vi "Configure Burst.vi"(0 "VISA resource name":refnum<visa-resource-name>, 1 "Start Phase (0.0 degrees)":dbl=0.002 min=0.0 max=360.0 format="%#.1g", 2 "Burst Cycle (0: N-Cycle)":u16(ring) items=["N-Cycle", "Infinite"], 3 "Number of Cycles (1)":i32=1, 4 "Burst Delay (1.352 μs)":dbl=1.352e-06, 5 "error in (no error)":errorcluster, 6 "Trigger Source (0: Internal)":u16(ring) items=["Internal", "External", "Manual"], 7 "External Trigger Condition (0: Rise)":u16(ring) items=["Rise", "Fall"], 8 "Enable Burst Mode (T:Enable)":bool=TRUE, 9 "Burst Period (0.01 s)":dbl=0.01 format="%#.3g", 10 "Channel (1:Channel 1)":i32(ring)=1 items=["Channel 1"=1, "Channel 2"=2], 11 "Trigger Out Mode (0: Off)":u16(ring) items=["Off", "Rise", "Fall"]) -> (14 "VISA resource name out":refnum<visa-resource-name>, 19 "error out":errorcluster)   [LabVIEW 2023, in "Siglent SDG X Series.lvlib"]
doc: "Configures and enables burst output mode.\n\nNote: Burst mode is not available for noise waveform."
uses:
  Siglent SDG X Series.lvlib
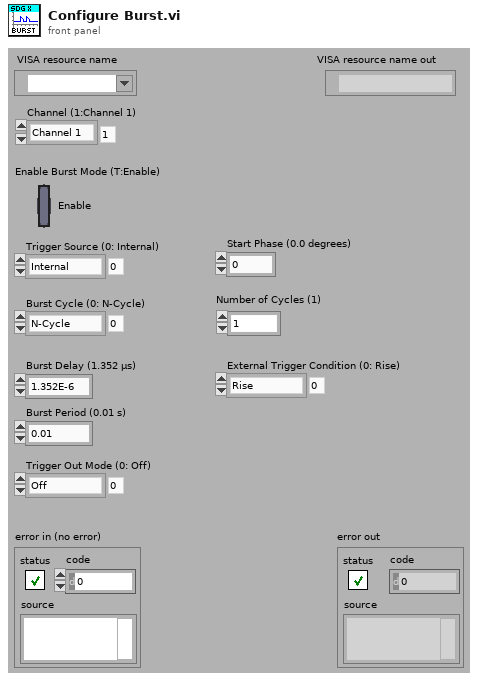
[diagram p1: front panel]
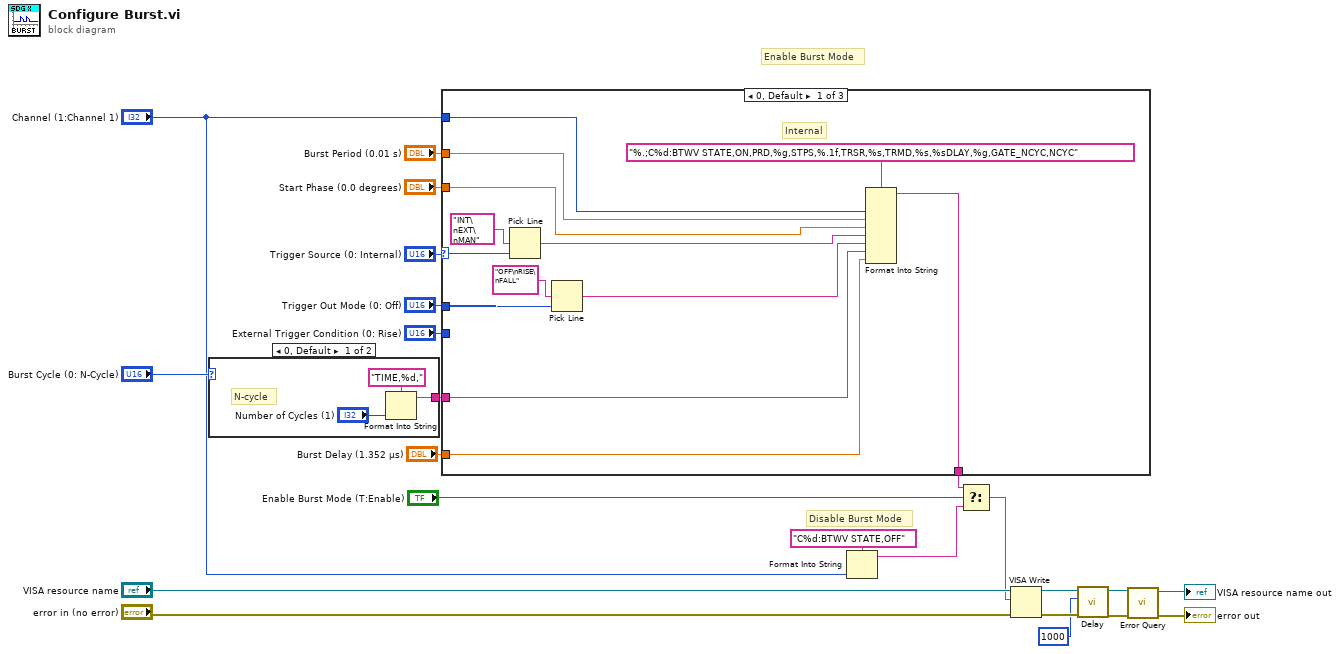
[diagram p0: block diagram]
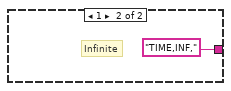
[diagram p2: hidden frame]
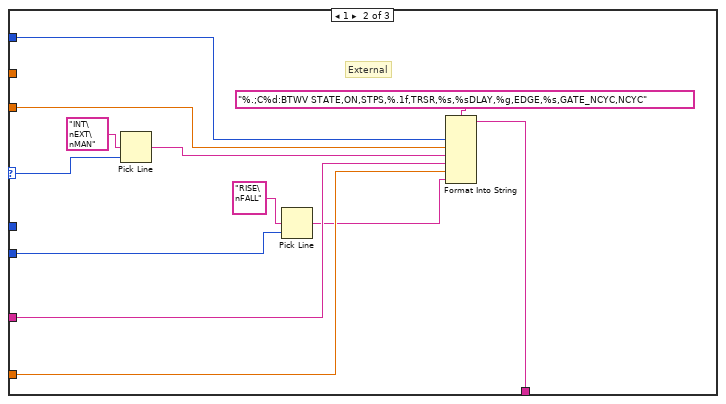
[diagram p3: hidden frame]
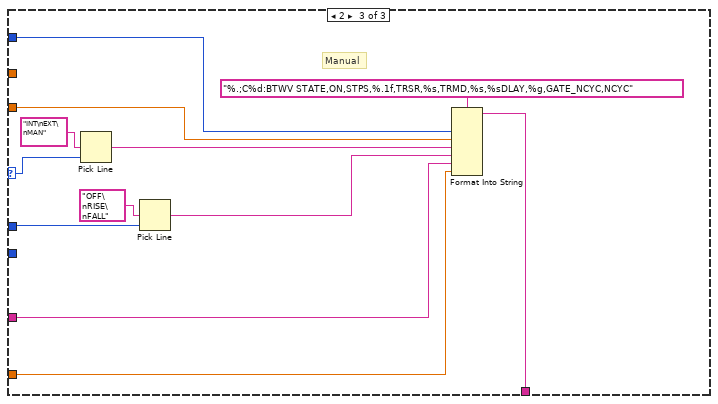
[diagram p4: hidden frame]
diagram:
  # "Disable Burst Mode"
  # "Enable Burst Mode"
  n1 = case shown="0, Default" "Burst Cycle (0: N-Cycle)" {
    tunnel: [w24 "TIME,INF,"] -> w13
    frame 0, Default {
      # "N-cycle"
      n2 = Format Into String(format string="TIME,%d,", "Number of Cycles (1)") -> (resulting string=w24:string)  [unwired: 2 in, 1 out]
    }
    frame 1 {
      # "Infinite"
    }
  }
  n3 = case shown="0, Default" "Trigger Source (0: Internal)" {
    selector: "Trigger Source (0: Internal)" -> [w37 w48 w61]
    tunnel: "Channel (1:Channel 1)" -> [w38 w50 w62]
    tunnel: "Burst Delay (1.352 μs)" -> [w33 w44 w53]
    tunnel: [w32 w42 w58] -> w12
    tunnel: "Trigger Out Mode (0: Off)" -> [w31 _ w59]
    tunnel: "Start Phase (0.0 degrees)" -> [w30 w49 w57]
    tunnel: w13 -> [w29 w45 w54]
    tunnel: "Burst Period (0.01 s)" -> [w28 _ _]
    tunnel: "External Trigger Condition (0: Rise)" -> [_ w41 _]
    frame 0, Default {
      # "Internal"
      n4 = Pick Line(multi-line string="INT\nEXT\nMAN", line index=w37) -> (output string=w35:string)  [unwired: 1 in]
      n5 = Pick Line(multi-line string="OFF\nRISE\nFALL", line index=w31) -> (output string=w34:string)  [unwired: 1 in]
      n6 = Format Into String(format string="%.;C%d:BTWV STATE,ON,PRD,%g,STPS,%.1f,TRSR,%s,TRMD,%s,%sDLAY,%g,GATE_NCYC,NCYC", w38, w28, w30, w35, w34, w29, w33) -> (resulting string=w32:string)  [unwired: 2 in, 1 out]
    }
    frame 1 {
      # "External"
      n7 = Pick Line(multi-line string="INT\nEXT\nMAN", line index=w48) -> (output string=w46:string)  [unwired: 1 in]
      n8 = Pick Line(multi-line string="RISE\nFALL", line index=w41) -> (output string=w43:string)  [unwired: 1 in]
      n9 = Format Into String(format string="%.;C%d:BTWV STATE,ON,STPS,%.1f,TRSR,%s,%sDLAY,%g,EDGE,%s,GATE_NCYC,NCYC", w50, w49, w46, w45, w44, w43) -> (resulting string=w42:string)  [unwired: 2 in, 1 out]
    }
    frame 2 {
      # "Manual"
      n10 = Pick Line(multi-line string="INT\nEXT\nMAN", line index=w61) -> (output string=w56:string)  [unwired: 1 in]
      n11 = Pick Line(multi-line string="OFF\nRISE\nFALL", line index=w59) -> (output string=w55:string)  [unwired: 1 in]
      n12 = Format Into String(format string="%.;C%d:BTWV STATE,ON,STPS,%.1f,TRSR,%s,TRMD,%s,%sDLAY,%g,GATE_NCYC,NCYC", w62, w57, w56, w55, w54, w53) -> (resulting string=w58:string)  [unwired: 2 in, 1 out]
    }
  }
  n13 = Format Into String(format string="C%d:BTWV STATE,OFF", "Channel (1:Channel 1)") -> (resulting string=w10:string)  [unwired: 2 in, 1 out]
  n14 = Select(t=w12, s="Enable Burst Mode (T:Enable)", f=w10) -> (s? t:f=w9:string)
  n15 = VISA Write(VISA resource name="VISA resource name", write buffer=w9, error in (no error)="error in (no error)") -> (VISA resource name out=w4:refnum<visa-resource-name>, error out=w5:errorcluster)  [unwired: 1 out]
  n16 = call "Delay.vi"("error in (no error)"=w5, "Delay Time (10)"=u32 1000, "VISA resource name"=w4) -> ("error out"=w2:errorcluster, "VISA resource name out"=w3:refnum<visa-resource-name>)  [unwired: 7 in]
  n17 = call "Error Query.vi"("error in (no error)"=w2, "VISA resource name"=w3) -> ("error out"=→"error out":errorcluster, "VISA resource name out"=→"VISA resource name out":refnum<visa-resource-name>)  [unwired: 6 in, 2 out]
